vi "BasicExample.vi"() -> ()   [LabVIEW 2013]
panel:
  in  "Timeout":dbl=0.1 format="%#_13g"
  out "TimedOut?":bool
  in  "stop":bool
  out "Status":i32 caption="Device Status"
  in  "Selector":T1(ring)
  out "Data":dbl[](graph)
  out "DeviceInfo":T2
  in  "Integration Time [s] (0.001)":dbl=0.001
  in  "resource name":refnum<visa-resource-name>
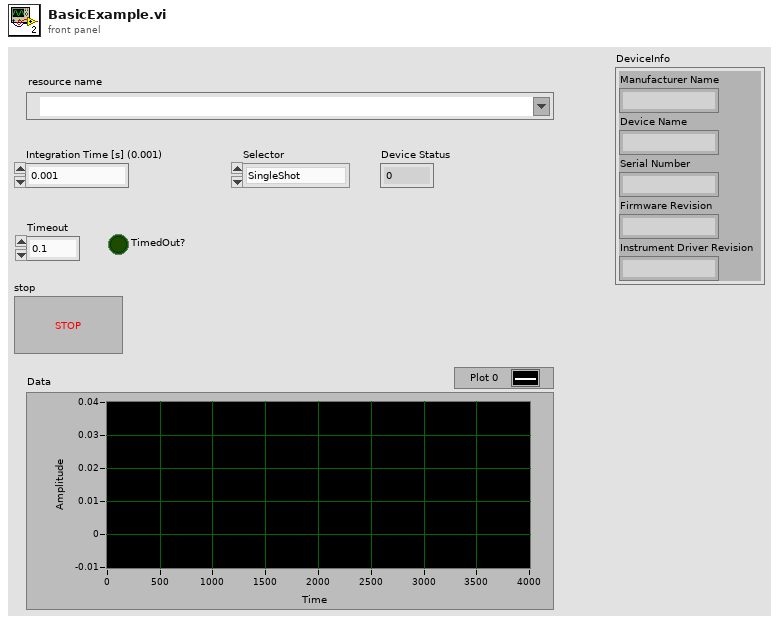
[diagram p1: front panel]
types:
  T1 = enum16{"SingleShot", "Continuos", "SingleTriggered", "ContinuosTriggered"}
  T2 = cluster{"Manufacturer Name":string, "Device Name":string, "Serial Number":string, "Firmware Revision":string, "Instrument Driver Revision":string}
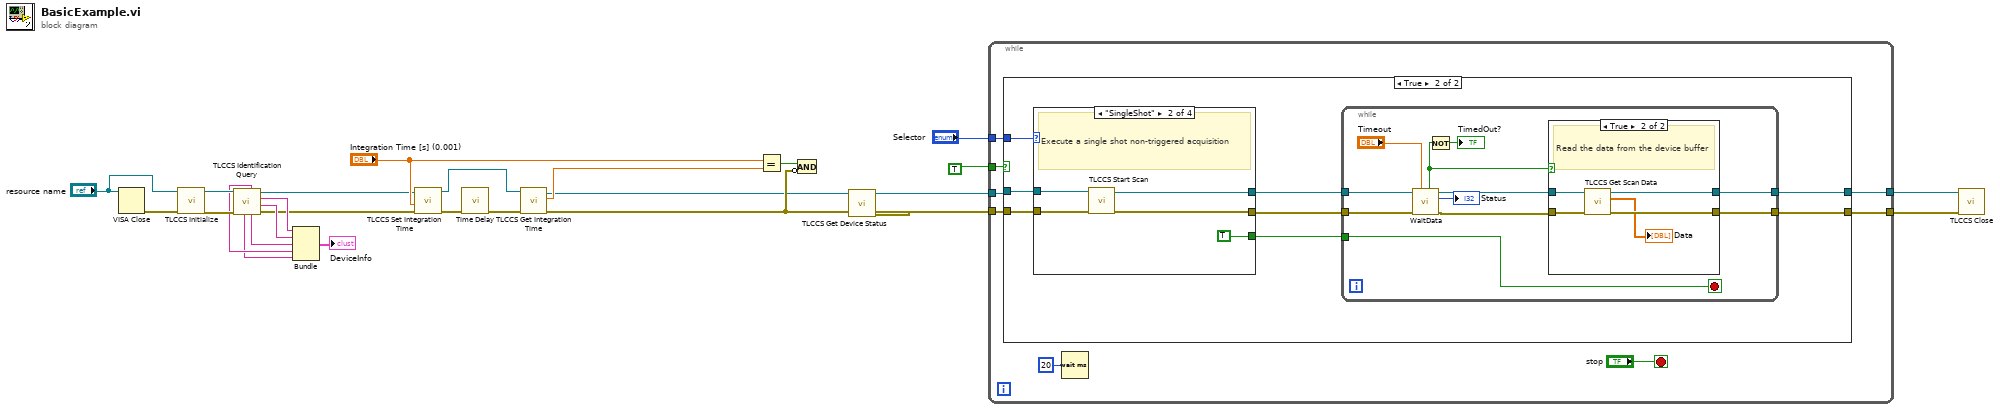
[diagram p0: block diagram]
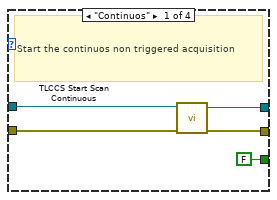
[diagram p4: hidden frame]
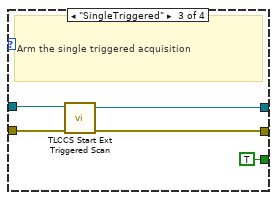
[diagram p5: hidden frame]
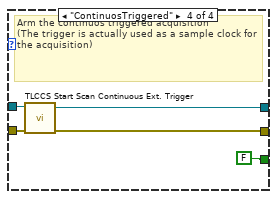
[diagram p6: hidden frame]
diagram:
  n1 = VISA Close(VISA resource name="resource name") -> (error out=w21:errorcluster)  [unwired: 1 in]
  n2 = call <instrlib>:"TLCCS Initialize.vi"("error in (no error)"=w21, "resource name"="resource name") -> ("error out"=w19:errorcluster, "instrument handle out"=w18:refnum<visa-resource-name>)  [unwired: 8 in]
  n3 = call <instrlib>:"TLCCS Identification Query.vi"("error in (no error)"=w19, "instrument handle"=w18) -> ("error out"=w4:errorcluster, "Device Name"=w16:string, "Manufacturer Name"=w17:string, "instrument handle out"=w3:refnum<visa-resource-name>, "Serial Number"=w15:string, "Firmware Revision"=w14:string, "Instrument Driver Revision"=w13:string)  [unwired: 3 in]
  n4 = Bundle("Manufacturer Name"=w17, "Device Name"=w16, "Serial Number"=w15, "Firmware Revision"=w14, "Instrument Driver Revision"=w13) -> (→"DeviceInfo":T2)  [unwired: 1 in]
  n5 = call <instrlib>:"TLCCS Set Integration Time.vi"("error in (no error)"=w4, "Integration Time [s] (0.001)"="Integration Time [s] (0.001)", "instrument handle"=w3) -> ("error out"=w26:errorcluster, "instrument handle out"=w24:refnum<visa-resource-name>)  [unwired: 7 in]
  n6 = call "Time Delay"("error in (no error)"=w26) -> ("error out"=w25:errorcluster)  [unwired: 10 in]
  n7 = call <instrlib>:"TLCCS Get Integration Time.vi"("error in (no error)"=w25, "instrument handle"=w24) -> ("error out"=w7:errorcluster, "Integration Time [s]"=w23:dbl, "instrument handle out"=w6:refnum<visa-resource-name>)  [unwired: 7 in]
  n8 = Equal?(x="Integration Time [s] (0.001)", y=w23) -> (x = y?=w11:bool)
  n9 = Compound Arithmetic op=AND(w11, invert w7) -> ()  [unwired: 1 out]
  n10 = call <instrlib>:"TLCCS Get Device Status.vi"("error in (no error)"=w7, "instrument handle"=w6) -> ("error out"=w5:errorcluster, "instrument handle out"=w2:refnum<visa-resource-name>)  [unwired: 7 in, 1 out]
  n11 = while {
    tunnel: TRUE -> [w34]
    tunnel: [w33] -> w10
    tunnel: [w32] -> w9
    tunnel: "Selector" -> [w31]
    tunnel: w2 -> [w30]
    tunnel: w5 -> [w29]
    stop <- "stop" stop-if-true
    n12 = case shown="True" w34 {
      tunnel: w30 -> [w35 w44]
      tunnel: w29 -> [w36 w43]
      tunnel: [w36 w38] -> w33
      tunnel: [w35 w39] -> w32
      tunnel: w31 -> [_ w42]
      frame False {
      }
      frame True {
        n13 = case shown="\"SingleShot\"" w42 {
          tunnel: [w65 w70 w75 w80] -> w40
          tunnel: [w64 w69 w74 w79] -> w37
          tunnel: w44 -> [w67 w72 w77 w82]
          tunnel: w43 -> [w66 w71 w76 w81]
          tunnel: [FALSE TRUE TRUE FALSE] -> w41
          frame "Continuos" {
            # "Start the continuos non triggered acquisition"
            n14 = call <instrlib>:"TLCCS Start Scan Continuous.vi"("error in (no error)"=w66, "instrument handle"=w67) -> ("error out"=w65:errorcluster, "instrument handle out"=w64:refnum<visa-resource-name>)  [unwired: 8 in]
          }
          frame "SingleShot" {
            # "Execute a single shot non-triggered acquisition"
            n15 = call <instrlib>:"TLCCS Start Scan.vi"("error in (no error)"=w71, "instrument handle"=w72) -> ("error out"=w70:errorcluster, "instrument handle out"=w69:refnum<visa-resource-name>)  [unwired: 8 in]
          }
          frame "SingleTriggered" {
            # "Arm the single triggered acquisition"
            n16 = call <instrlib>:"TLCCS Start Ext Triggered Scan.vi"("error in (no error)"=w76, "instrument handle"=w77) -> ("error out"=w75:errorcluster, "instrument handle out"=w74:refnum<visa-resource-name>)  [unwired: 8 in]
          }
          frame "ContinuosTriggered" {
            # "Arm the continuos triggered acquisition\n(The trigger is actually used as a sample clock for the acquisition)"
            n17 = call <instrlib>:"TLCCS Start Scan Continuous Ext. Trigger.vi"("error in (no error)"=w81, "instrument handle"=w82) -> ("error out"=w80:errorcluster, "instrument handle out"=w79:refnum<visa-resource-name>)  [unwired: 8 in]
          }
        }
        n18 = while {
          tunnel: w41 -> [w45]
          tunnel: w40 -> [w55]
          tunnel: [w54] -> w39
          tunnel: [w53] -> w38
          tunnel: w37 -> [w46]
          stop <- w45 stop-if-true
          n19 = call "WaitData.vi"("error in (no error)"=w55, "Timeout"="Timeout", "VISA Refnum in"=w46) -> ("error out"=w50:errorcluster, "Device Status"=→"Status":i32, "VISA Refnum out"=w51:refnum<visa-resource-name>, "OK?"=w48:bool)  [unwired: 5 in]
          n20 = Not(x=w48) -> (.not. x?=→"TimedOut?":bool)
          n21 = case shown="True" w48 {
            tunnel: [w56 w62] -> w53
            tunnel: [w57 w61] -> w54
            tunnel: w50 -> [w56 w59]
            tunnel: w51 -> [w57 w58]
            frame False {
            }
            frame True {
              # "Read the data from the device buffer"
              n22 = call <instrlib>:"TLCCS Get Scan Data.vi"("error in (no error)"=w59, "instrument handle"=w58) -> ("error out"=w62:errorcluster, "Data"=→"Data":dbl[], "instrument handle out"=w61:refnum<visa-resource-name>)  [unwired: 7 in]
            }
          }
        }
      }
    }
    n23 = Wait (ms)(milliseconds to wait=u32 20) -> ()  [unwired: 1 out]
  }
  n24 = call <instrlib>:"TLCCS Close.vi"("error in (no error)"=w10, "instrument handle"=w9) -> ()  [unwired: 9 in, 1 out]
